vi "Test Envelope Plot.vi"() -> ()   [LabVIEW 2020, in "Moving Ripple Noise.lvclass"]
uses:
  Moving Ripple Noise.lvclass
  Serialized.ctl
  Moving Ripple Noise.lvclass/Moving Ripple Noise.ctl
panel:
  in  "Serialized":T1={"Fmin (Hz)"=250.0, "Fmax (Hz)"=8000.0, "Comp/oct"=12, "Depth (0-1)"=0.9, "Density (cyc/oct)"=2.0, "Velocity (Hz)"=1.0, "Phase (0-1)"=0.0}
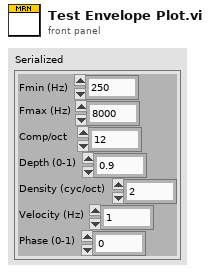
[diagram p1: front panel]
types:
  T1 = typedef "Moving Ripple Noise.lvclass/Serialized.ctl" = cluster{"Fmin (Hz)":dbl, "Fmax (Hz)":dbl, "Comp/oct":i32, "Depth (0-1)":dbl, "Density (cyc/oct)":dbl, "Velocity (Hz)":dbl, "Phase (0-1)":dbl}
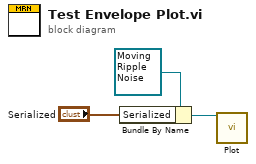
[diagram p0: block diagram]
diagram:
  n1 = Bundle By Name(cluster=refnum<class "Moving Ripple Noise.lvclass"> refnum ("MRN in"), "Serialized"="Serialized") -> (w1:refnum<class "Moving Ripple Noise.lvclass">)
  n2 = call "Plot.vi"("MRN in"=w1) -> ()  [unwired: 13 in, 2 out]
